vi "Create.vi"(3 "Parent Name":string) -> (1 "DataProc Identity out":refnum<class "DataProc Identity.lvclass">)   [LabVIEW 2020, in "VolatusData.lvlib" / "DataProc Identity.lvclass"]
uses:
  DataProc Identity.lvclass
  DataProc Identity.lvclass/DataProc Identity.ctl
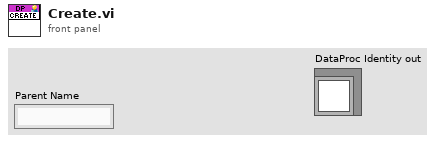
[diagram p1: front panel]
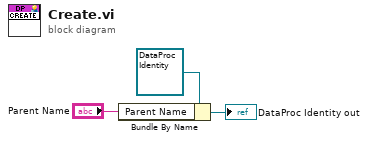
[diagram p0: block diagram]
diagram:
  n1 = Bundle By Name(cluster=refnum<class "DataProc Identity.lvclass"> refnum ("DataProc Identity in"), "Parent Name"="Parent Name") -> (→"DataProc Identity out":refnum<class "DataProc Identity.lvclass">)
